vi "SCTL Sector Accumulation Pipelined V3.vi"() -> (3 "New Data?":bool)   [LabVIEW 2013]
uses:
  FPGA/Sector/Accumulate/Accumulated Count Array Fixed Point.ctl
  <vilib>/rvi/Emulation/niFpgaSctlEmulationGetInTimedLoop.vi
  <vilib>/rvi/Memory/Memory_Emulation/niFpgaMemoryEmulationReadFromVariant.vi
  <vilib>/rvi/Memory/Memory_Emulation/niFpgaMemoryEmulationWriteToVariant.vi
  <vilib>/rvi/DataTransferAndStorage/Container/Common/niFpgaContainerGetUniqueNameForEmu.vi
  <vilib>/rvi/FIFO/Fifo_Resource/nirvififoEmulationSetSize.vi
  <vilib>/rvi/Emulation/niFpgaSctlEmulationFifoFullMgr.vi
  <vilib>/rvi/errors/niFpgaSetErrorForExecOnDevCompSimple.vi
  <vilib>/rvi/eio/common/nirviEmuReportErrorAndStop.vi
  <vilib>/rvi/Emulation/niFpgaSctlEmulationResourceMgr.vi
  <vilib>/rvi/Memory/Memory_Emulation/nirvimemoryFastEmulation.vi
  <vilib>/rvi/Memory/Memory_Emulation/nirvimemoryEmulation.vi
  <vilib>/rvi/DataTransferAndStorage/Container/XNode/niFpgaContainer.xnode
  <vilib>/rvi/FIFO/Fifo_Resource/nirvififoEmulationRead.vi
panel:
  out "Accummulated":T1(array[cluster])
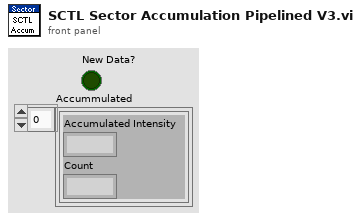
[diagram p1: front panel]
types:
  T1 = cluster{"Accumulated Intensity":fxp<+,20,20>, "Count":fxp<+,12,12>}[]
  T2 = cluster{"Accumulated Intensity":fxp<+,8,8>, "Count":fxp<+,1,1>}
  T3 = typedef "Accumulated Count Array Fixed Point.ctl" = cluster{"Accumulated Intensity":fxp<+,20,20>, "Count":fxp<+,12,12>}[]
  T4 = cluster{"Accumulated Intensity":fxp<+,21,21>, "Count":fxp<+,13,13>}[]
  T5 = cluster{"Accumulated Intensity":fxp<+,22,22>, "Count":fxp<+,14,14>}[]
  T6 = cluster{"Accumulated Intensity":fxp<+,23,23>, "Count":fxp<+,15,15>}[]
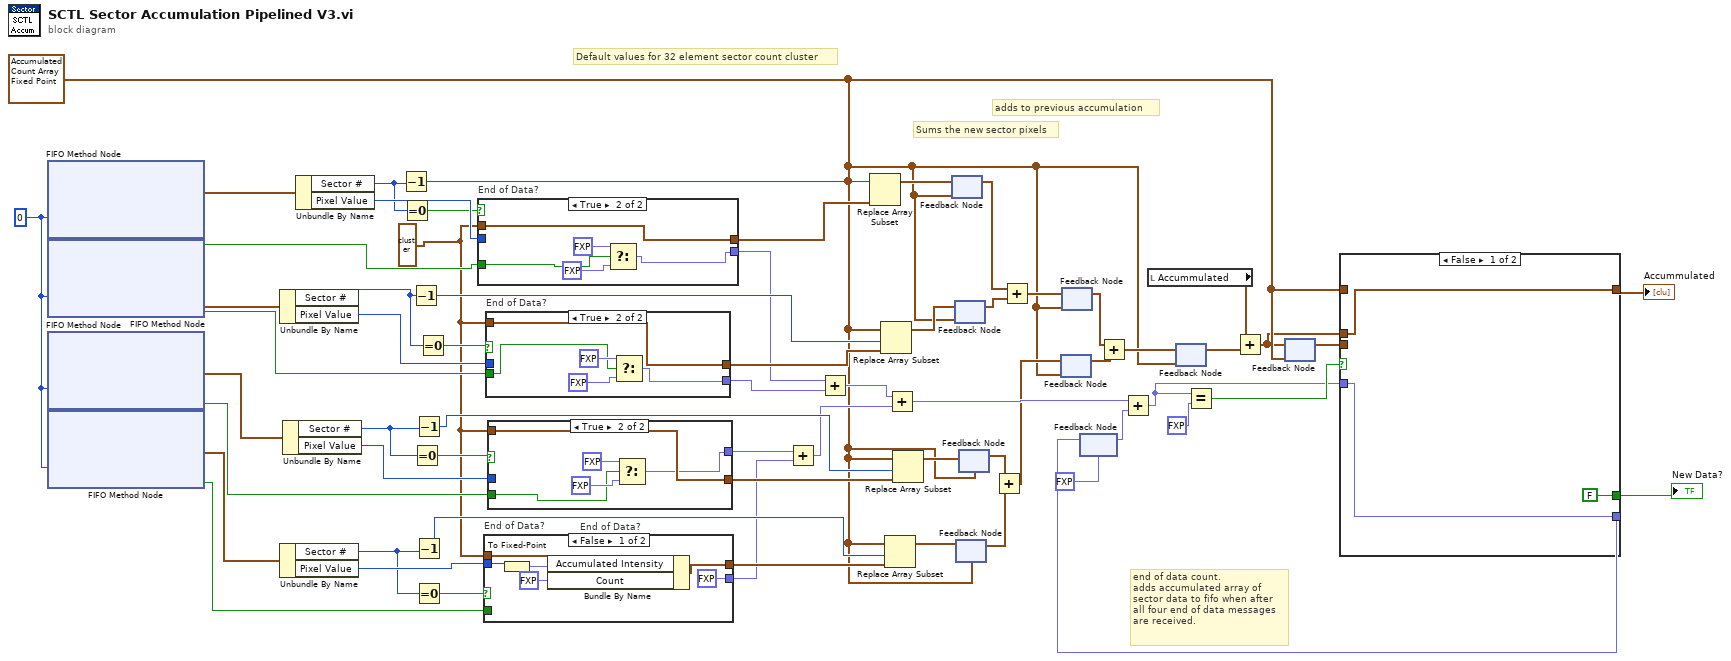
[diagram p0: block diagram]
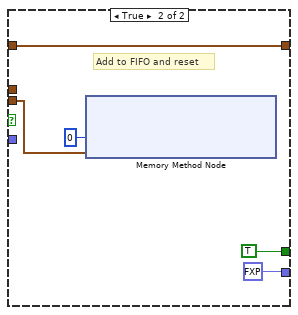
[diagram p2: hidden frame]
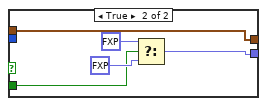
[diagram p3: hidden frame]
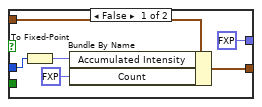
[diagram p4: hidden frame]
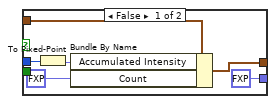
[diagram p5: hidden frame]
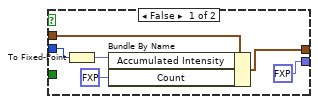
[diagram p6: hidden frame]
diagram:
  w24 = T2 {"Accumulated Intensity"=0.0, "Count"=0.0} ("Accumulated Sector Cluster")
  w6 = T3 [{"Accumulated Intensity"=0.0, "Count"=0.0}, {"Accumulated Intensity"=0.0, "Count"=0.0}, {"Accumulated Intensity"=0.0, "Count"=0.0}, {"Accumulated Intensity"=0.0, "Count"=0.0}, {"Accumulated Intensity"=0.0, "Count"=0.0}, {"Accumulated Intensity"=0.0, "Count"=0.0}, {"Accumulated Intensity"=0.0, "Count"=0.0}, {"Accumulated Intensity"=0.0, "Count"=0.0}, {"Accumulated Intensity"=0.0, "Count"=0.0}, {"Accumulated Intensity"=0.0, "Count"=0.0}, {"Accumulated Intensity"=0.0, "Count"=0.0}, {"Accumulated Intensity"=0.0, "Count"=0.0}, {"Accumulated Intensity"=0.0, "Count"=0.0}, {"Accumulated Intensity"=0.0, "Count"=0.0}, {"Accumulated Intensity"=0.0, "Count"=0.0}, {"Accumulated Intensity"=0.0, "Count"=0.0}, {"Accumulated Intensity"=0.0, "Count"=0.0}, {"Accumulated Intensity"=0.0, "Count"=0.0}, {"Accumulated Intensity"=0.0, "Count"=0.0}, {"Accumulated Intensity"=0.0, "Count"=0.0}, {"Accumulated Intensity"=0.0, "Count"=0.0}, {"Accumulated Intensity"=0.0, "Count"=0.0}, {"Accumulated Intensity"=0.0, "Count"=0.0}, {"Accumulated Intensity"=0.0, "Count"=0.0}, {"Accumulated Intensity"=0.0, "Count"=0.0}, {"Accumulated Intensity"=0.0, "Count"=0.0}, {"Accumulated Intensity"=0.0, "Count"=0.0}, {"Accumulated Intensity"=0.0, "Count"=0.0}, {"Accumulated Intensity"=0.0, "Count"=0.0}, {"Accumulated Intensity"=0.0, "Count"=0.0}, {"Accumulated Intensity"=0.0, "Count"=0.0}, {"Accumulated Intensity"=0.0, "Count"=0.0}] ("Test Accumulated Array")
  w63 = 0 ("Timeout")
  # "end of data count.\nadds accumulated array of\nsector data to fifo when after\nall four end of data messages\nare received."
  # "adds to previous accumulation"
  # "Sums the new sector pixels"
  # "Default values for 32 element sector count cluster"
  n1 = xnode ("FIFO Method Node")("Timeout"=w63) -> ("Element"=w39:cluster{"Sector #":u8, "Pixel Value":u8}, "Timed Out?"=w35:bool)  [unwired: 1 in, 1 out]
  n2 = xnode ("FIFO Method Node")("Timeout"=w63) -> ("Element"=w38:cluster{"Sector #":u8, "Pixel Value":u8}, "Timed Out?"=w34:bool)  [unwired: 1 in, 1 out]
  n3 = xnode ("FIFO Method Node")("Timeout"=w63) -> ("Element"=w37:cluster{"Sector #":u8, "Pixel Value":u8}, "Timed Out?"=w33:bool)  [unwired: 1 in, 1 out]
  n4 = xnode ("FIFO Method Node")("Timeout"=w63) -> ("Element"=w36:cluster{"Sector #":u8, "Pixel Value":u8}, "Timed Out?"=w32:bool)  [unwired: 1 in, 1 out]
  n5 = Unbundle By Name(w38) -> ("Sector #"=w49:u8, "Pixel Value"=w59:u8)
  n6 = Unbundle By Name(w36) -> ("Sector #"=w45:u8, "Pixel Value"=w53:u8)
  n7 = Unbundle By Name(w37) -> ("Sector #"=w47:u8, "Pixel Value"=w56:u8)
  n8 = Unbundle By Name(w39) -> ("Sector #"=w51:u8, "Pixel Value"=w61:u8)
  n9 = Decrement(x=w51) -> (x-1=w62:u8)
  n10 = Equal To 0?(x=w51) -> (x = 0?=w50:bool)
  n11 = Decrement(x=w49) -> (x-1=w58:u8)
  n12 = Equal To 0?(x=w47) -> (x = 0?=w46:bool)
  n13 = Decrement(x=w47) -> (x-1=w40:u8)
  n14 = Decrement(x=w45) -> (x-1=w55:u8)
  n15 = Equal To 0?(x=w45) -> (x = 0?=w44:bool)
  n16 = Equal To 0?(x=w49) -> (x = 0?=w48:bool)
  n17 = case "End of Data?" shown="True" w50 {
    tunnel: w61 -> [w65 _]
    tunnel: [w69 w74] -> w60
    tunnel: w24 -> [w68 w74]
    tunnel: [fxp<+,1,1> 0.0 w70] -> w31
    tunnel: w35 -> [_ w73]
    frame False {
      n18 = To Fixed-Point(number=w65) -> (fixed-point=w64:fxp<+,8,8>)  [unwired: 1 in]
      n19 = Bundle By Name(cluster=w68, "Accumulated Intensity"=w64, "Count"=fxp<+,1,1> 1.0) -> (w69:T2)
    }
    frame True {
      n20 = Select(t=fxp<+,1,1> 0.0, s=w73, f=fxp<+,1,1> 1.0) -> (s? t:f=w70:fxp<+,1,1>)
    }
  }
  n21 = case "End of Data?" shown="False" w44 {
    tunnel: [w80 w85] -> w54
    tunnel: w24 -> [w79 w85]
    tunnel: w53 -> [w75 _]
    tunnel: [fxp<+,1,1> 0.0 w81] -> w28
    tunnel: w32 -> [_ w82]
    frame False {
      n22 = To Fixed-Point(number=w75) -> (fixed-point=w76:fxp<+,8,8>)  [unwired: 1 in]
      n23 = Bundle By Name(cluster=w79, "Accumulated Intensity"=w76, "Count"=fxp<+,1,1> 1.0) -> (w80:T2)
    }
    frame True {
      n24 = Select(t=fxp<+,1,1> 0.0, s=w82, f=fxp<+,1,1> 1.0) -> (s? t:f=w81:fxp<+,1,1>)
    }
  }
  n25 = case "End of Data?" shown="True" w48 {
    tunnel: w59 -> [w87 _]
    tunnel: w24 -> [w91 w96]
    tunnel: [w90 w96] -> w52
    tunnel: [fxp<+,1,1> 0.0 w92] -> w30
    tunnel: w34 -> [_ w93]
    frame False {
      n26 = To Fixed-Point(number=w87) -> (fixed-point=w86:fxp<+,8,8>)  [unwired: 1 in]
      n27 = Bundle By Name(cluster=w91, "Accumulated Intensity"=w86, "Count"=fxp<+,1,1> 1.0) -> (w90:T2)
    }
    frame True {
      n28 = Select(t=fxp<+,1,1> 0.0, s=w93, f=fxp<+,1,1> 1.0) -> (s? t:f=w92:fxp<+,1,1>)
    }
  }
  n29 = case "End of Data?" shown="True" w46 {
    tunnel: [w102 w107] -> w57
    tunnel: w56 -> [w98 _]
    tunnel: w24 -> [w101 w107]
    tunnel: [fxp<+,1,1> 0.0 w103] -> w29
    tunnel: w33 -> [_ w104]
    frame False {
      n30 = To Fixed-Point(number=w98) -> (fixed-point=w97:fxp<+,8,8>)  [unwired: 1 in]
      n31 = Bundle By Name(cluster=w101, "Accumulated Intensity"=w97, "Count"=fxp<+,1,1> 1.0) -> (w102:T2)
    }
    frame True {
      n32 = Select(t=fxp<+,1,1> 0.0, s=w104, f=fxp<+,1,1> 1.0) -> (s? t:f=w103:fxp<+,1,1>)
    }
  }
  n33 = Add(x=w29, y=w28) -> (x+y=w26:fxp<+,2,2>)
  n34 = Add(x=w31, y=w30) -> (x+y=w27:fxp<+,2,2>)
  n35 = Replace Array Subset(array=w6, new element=w60, index=w62) -> (w21:T3)
  n36 = Replace Array Subset(array=w6, new element=w52, index=w58) -> (w19:T3)
  n37 = Replace Array Subset(array=w6, new element=w54, index=w55) -> (w15:T3)
  n38 = Add(x=w27, y=w26) -> (x+y=w25:fxp<+,3,3>)
  n39 = Replace Array Subset(array=w6, new element=w57, index=w40) -> (w17:T3)
  n40 = feedback #1(w6) -> (w20:T3)
  n41 = feedback-in #1(w21) -> ()
  n42 = feedback #2(w6) -> (w18:T3)
  n43 = feedback-in #2(w19) -> ()
  n44 = feedback #3(w6) -> (w14:T3)
  n45 = feedback-in #3(w15) -> ()
  n46 = feedback #4(w6) -> (w16:T3)
  n47 = feedback-in #4(w17) -> ()
  n48 = Add(x=w16, y=w14) -> (x+y=w11:T4)
  n49 = Add(x=w20, y=w18) -> (x+y=w13:T4)
  n50 = feedback #5(w6) -> (w10:T4)
  n51 = feedback-in #5(w11) -> ()
  n52 = feedback #6(w6) -> (w12:T4)
  n53 = feedback-in #6(w13) -> ()
  n54 = feedback #7(fxp<+,3,3> 0.0 ("y")) -> (w2:fxp<+,3,3>)
  n55 = Add(x=w12, y=w10) -> (x+y=w9:T5)
  n56 = Add(x=w25, y=w2) -> (x+y=w1:fxp<+,3,3>)
  n57 = local read "Accummulated"() -> (w23:T1)
  n58 = feedback #8(w6) -> (w8:T5)
  n59 = feedback-in #8(w9) -> ()
  n60 = Equal?(x=w1, y=fxp<+,3,3> 4.0) -> (x = y?=w42:bool)
  n61 = Add(x=w23, y=w8) -> (x+y=w5:T6)
  n62 = feedback #9(w6) -> (w7:T6)
  n63 = feedback-in #9(w5) -> ()
  n64 = case shown="False" w42 {
    tunnel: w7 -> [_ w111]
    tunnel: [w109 fxp<+,3,3> 0.0] -> w3
    tunnel: w1 -> [w109 _]
    tunnel: w6 -> [_ w112]
    tunnel: [FALSE ("New Data?") TRUE ("New Data?")] -> w41
    tunnel: [w108 w112] -> w22
    tunnel: w5 -> [w108 _]
    frame False {
    }
    frame True {
      # "Add to FIFO and reset"
      n65 = xnode ("Memory Method Node")("Address"=u32 0, "Data"=w111) -> ()  [unwired: 1 in, 1 out]
    }
  }
  "New Data?" <- w41
  "Accummulated" <- w22
  n66 = feedback-in #7(w3) -> ()
